vi "PPS_TDK_Lambda.vi"(0 "VISA":refnum<visa-resource-name>="COM1", 1 "GEN Addr":i16=6, 2 "BAUD":u16(ring)=3 items=["1200", "2400", "4800", "9600", "19200"], 5 "Voltage Limit":dbl format="%.4f", 7 "Current Limit":dbl format="%.4f", 11 "error":errorcluster, 12 "Reset (T)":bool=TRUE, 13 "Output On (T)":bool=TRUE, 14 "Settle (0 mS)":u32=1000) -> (4 "VISA out":refnum<visa-resource-name>, 6 "Output Voltage":dbl format="%.4f", 8 "Output Current":dbl format="%.4f", 15 "error out":errorcluster)   [LabVIEW 2016]
doc: "This is a simple VI to demonstrate the operation of the Lambda Genesys series DC Power Supply using the serial RS-232 or RS-485 port. This VI programs the output voltage and current, turns the output on and measures the output voltage and current.\n\nThis VI may be run as a stand-alone program if the required controls are set to the correct COM port and the power supply's address and BAUD rate. This VI may also be called as a sub-VI."
panel:
  out "code (hex)":i32 format="%.0x"
  # "Lambda Genesys \nSerial Port\n  DC Power Supplies"
  # "Getting Started:\nConfigure and Read Once"
  # "Right-Click any control\nto see it's \"Description\""
  # "WAIT"
  # "MEASURE"
  # "CONFIGURE"
  # "Right-Click to\nexplain error"
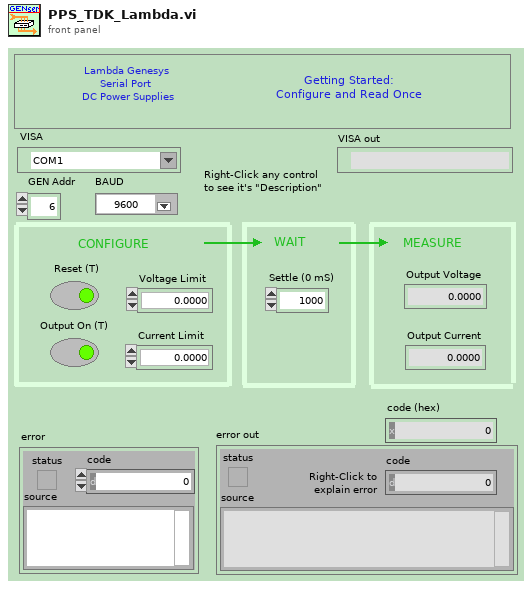
[diagram p1: front panel]
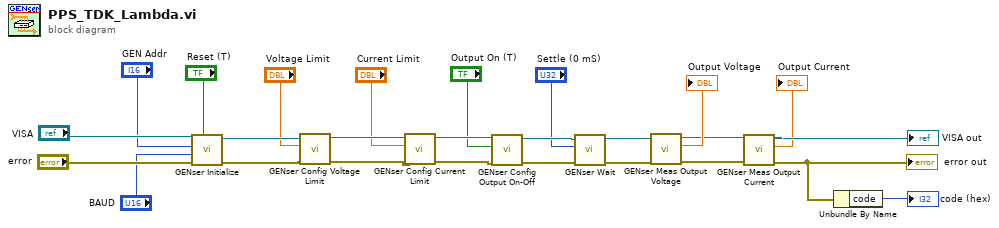
[diagram p0: block diagram]
diagram:
  n1 = call <instrlib>:"GENser Initialize.vi"("Reset (T)"="Reset (T)", "error in (no error)"="error", "BAUD"="BAUD", "GEN Addr"="GEN Addr", "VISA name"="VISA") -> ("error out"=w23:errorcluster, "VISA out"=w24:refnum<visa-resource-name>)  [unwired: 5 in]
  n2 = call <instrlib>:"GENser Config Voltage Limit.vi"("error"=w23, "Volt Limit"="Voltage Limit", "VISA"=w24) -> ("error out"=w20:errorcluster, "VISA out"=w21:refnum<visa-resource-name>)  [unwired: 7 in]
  n3 = call <instrlib>:"GENser Config Current Limit.vi"("error"=w20, "Current Limit"="Current Limit", "VISA"=w21) -> ("error out"=w17:errorcluster, "VISA out"=w18:refnum<visa-resource-name>)  [unwired: 7 in]
  n4 = call <instrlib>:"GENser Config Output On-Off.vi"("error"=w17, "Output ON"="Output On (T)", "VISA"=w18) -> ("error out"=w15:errorcluster, "VISA out"=w16:refnum<visa-resource-name>)  [unwired: 7 in]
  n5 = call <instrlib>:"GENser Wait.vi"("error"=w15, "Delay (20 mS)"="Settle (0 mS)", "VISA"=w16) -> ("error out"=w12:errorcluster, "VISA out"=w13:refnum<visa-resource-name>)  [unwired: 7 in]
  n6 = call <instrlib>:"GENser Meas Output Voltage.vi"("error"=w12, "VISA"=w13) -> ("error out"=w9:errorcluster, "Output Voltage"=→"Output Voltage":dbl, "VISA out"=w10:refnum<visa-resource-name>)  [unwired: 7 in]
  n7 = call <instrlib>:"GENser Meas Output Current.vi"("error"=w9, "VISA"=w10) -> ("error out"=w6:errorcluster, "Output Current"=→"Output Current":dbl, "VISA out"=→"VISA out":refnum<visa-resource-name>)  [unwired: 7 in]
  "error out" <- w6
  n8 = Unbundle By Name(w6) -> ("code"=→"code (hex)":i32)
